vi "LoginInteraction.vi"(10 "LoginStatus":T1, 11 "DataIn":T2={"Quem Joga"="", "Tabuleiro"={"(0,0)"="", "(1,0)"="", "(0,1)"="", "(1,1)"="", "(2,0)"="", "(1,2)"="", "(2,2)"="", "(0,2)"="", "(2,1) "=""}, "GameOption"=enum."Multiplayer local", "Turno"=FALSE, "Player"="", "Player 1"="", "Player 2"="", "Dificuldade"=enum."Easy", "Table"=[], "Row"=0, "Aceitar Convite"=FALSE, "Inviter line"=0, "diretório"=path "", "Logout - panel close"=FALSE, "StartGame"=FALSE, "MatchData.lvclass"=refnum, "GameMode"=enum."Single Easy", "Level State"=FALSE}) -> (2 "Next state":string, 3 "DataOut":T2={"Quem Joga"="", "Tabuleiro"={"(0,0)"="", "(1,0)"="", "(0,1)"="", "(1,1)"="", "(2,0)"="", "(1,2)"="", "(2,2)"="", "(0,2)"="", "(2,1) "=""}, "GameOption"=enum."Multiplayer local", "Turno"=FALSE, "Player"="", "Player 1"="", "Player 2"="", "Dificuldade"=enum."Easy", "Table"=[], "Row"=0, "Aceitar Convite"=FALSE, "Inviter line"=0, "diretório"=path "", "Logout - panel close"=FALSE, "StartGame"=FALSE, "MatchData.lvclass"=refnum, "GameMode"=enum."Single Easy", "Level State"=FALSE})   [LabVIEW 2018]
doc: "SubVI criada para realizar operações de leitura e escrita em arquivo"
uses:
  controls/DataIn.ctl
  MatchDataClasses/MatchData/MatchData.lvclass
  controls/Tabuleiro.ctl
  controls/Table.ctl
  controls/LoginStatus.ctl
  <vilib>/Utility/file.llb/Read Delimited Spreadsheet (string).vi
  <vilib>/Utility/file.llb/Write Delimited Spreadsheet (string).vi
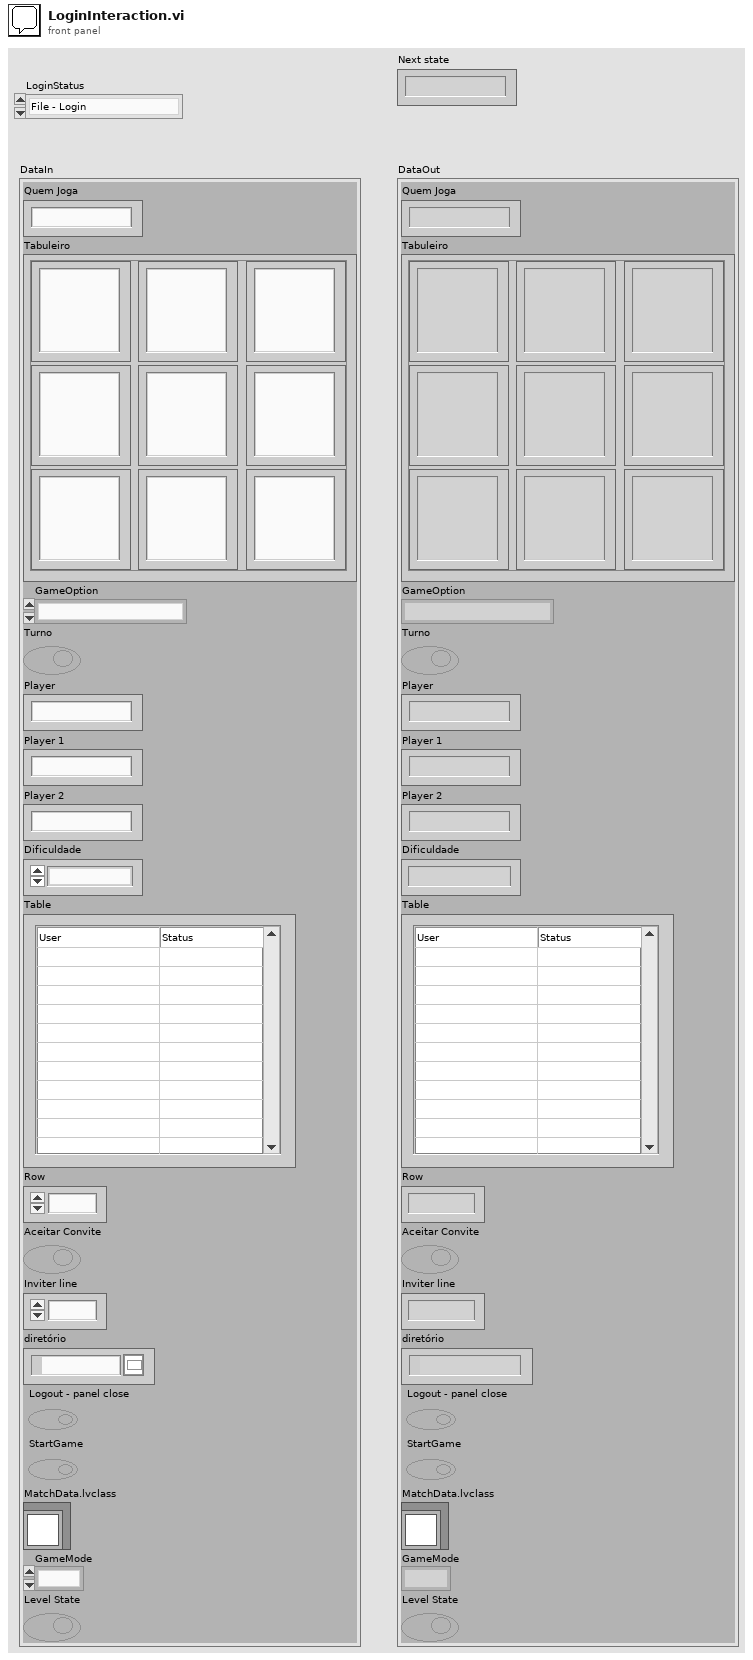
[diagram p1: front panel]
types:
  T1 = typedef "LoginStatus.ctl" = enum16{"File - Login", "File - Logout", "File - TableRefresh"}
  T2 = typedef "DataIn.ctl" = cluster{"Quem Joga":string, "Tabuleiro":T3, "GameOption":enum16{"Single Player", "Multiplayer local", "Multiplayer remoto", "Wait for Event", "Initialize", "Stop"}, "Turno":bool, "Player":string, "Player 1":string, "Player 2":string, "Dificuldade":enum16{"Easy", "Medium", "Hard"}, "Table":T4, "Row":u32, "Aceitar Convite":bool, "Inviter line":u32, "diretório":path, "Logout - panel close":bool, "StartGame":bool, "MatchData.lvclass":refnum<class "MatchData.lvclass">, "GameMode":enum16{"Single Easy", "Single Medium", "Single Hard", "Local", "Remote"}, "Level State":bool}
  T3 = typedef "Tabuleiro.ctl" = cluster{"(0,0)":string, "(1,0)":string, "(0,1)":string, "(1,1)":string, "(2,0)":string, "(1,2)":string, "(2,2)":string, "(0,2)":string, "(2,1) ":string}
  T4 = typedef "Table.ctl" = string[][]
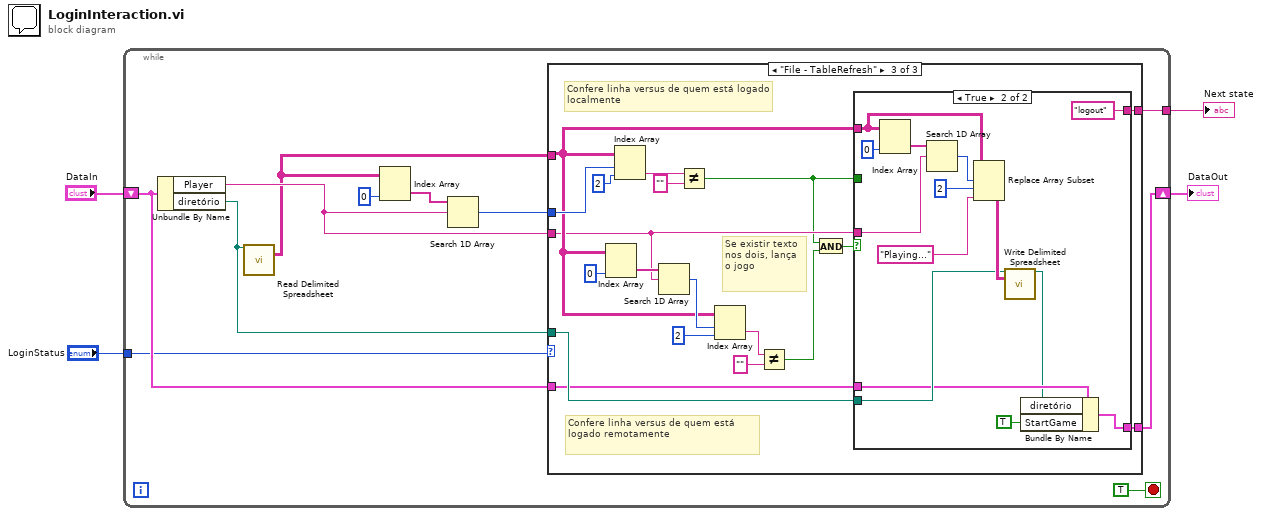
[diagram p0: block diagram]
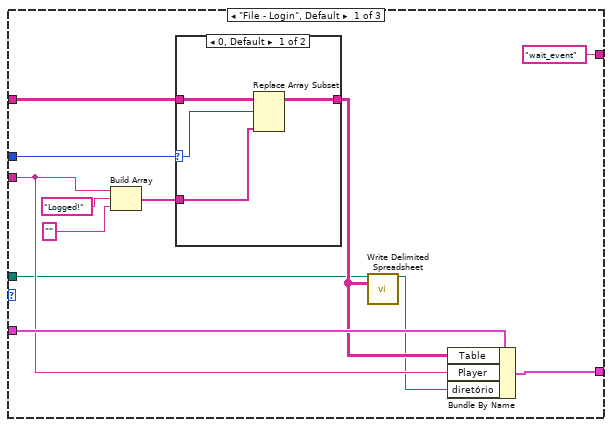
[diagram p2: hidden frame]
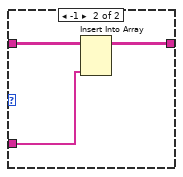
[diagram p3: hidden frame]
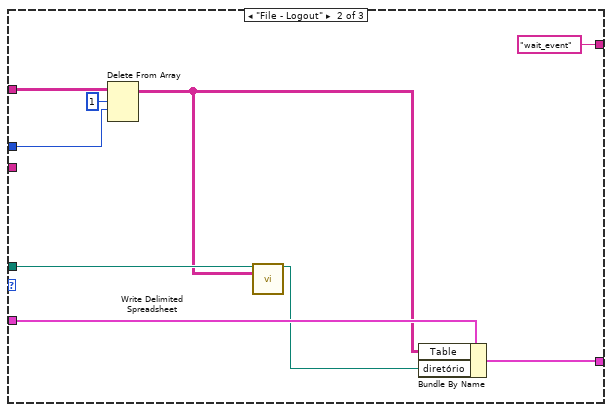
[diagram p4: hidden frame]
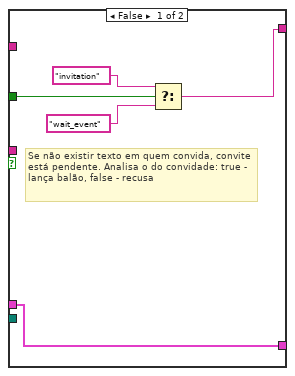
[diagram p5: hidden frame]
diagram:
  n1 = while {
    tunnel: "LoginStatus" -> [w7]
    shift-right: [w8] -> w3
    shift-left: "DataIn" -> [w9]
    tunnel: [w5] -> w1
    stop <- TRUE stop-if-true
    n2 = Unbundle By Name(w9) -> ("Player"=w12:string, "diretório"=w10:path)
    n3 = call-poly <vilib>:"Read Delimited Spreadsheet.vi"("file path (dialog if empty)"=w10) -> ("all rows"=w11:string[][])  [unwired: 9 in, 5 out]
    n4 = Index Array(array=w11, index (col)=0 ("disabled index (col)")) -> (element=w14:string[])  [unwired: 1 in]
    n5 = Search 1D Array(1D array=w14, element=w12) -> (index of element=w13:i32)  [unwired: 1 in]
    n6 = case shown="\"File - TableRefresh\"" w7 {
      tunnel: w13 -> [w25 w42 w62]
      tunnel: w12 -> [w20 _ w49]
      tunnel: w11 -> [w24 w43 w50]
      tunnel: w10 -> [w19 w40 w48]
      tunnel: w9 -> [w22 w39 w47]
      tunnel: [w18 w36 w46] -> w8
      tunnel: ["wait_event" "wait_event" w44] -> w5
      frame "File - Login", Default {
        n7 = Build Array(w20, "Logged!" ("string"), "" ("string")) -> (w23:string[])
        n8 = case shown="0, Default" w25 {
          selector: w25 -> [w30 _]
          tunnel: w23 -> [w28 w32]
          tunnel: w24 -> [w31 w34]
          tunnel: [w29 w33] -> w21
          frame 0, Default {
            n9 = Replace Array Subset(array=w31, new element=w28, index (row)=w30) -> (w29:string[][])  [unwired: 1 in]
          }
          frame -1 {
            n10 = Insert Into Array(array=w34, new element=w32) -> (w33:string[][])  [unwired: 2 in]
          }
        }
        n11 = call-poly <vilib>:"Write Delimited Spreadsheet.vi"("file path (dialog if empty)"=w19, "2D data"=w21) -> ("new file path (Not A Path if cancelled)"=w17:path)  [unwired: 12 in, 1 out]
        n12 = Bundle By Name(cluster=w22, "Table"=w21, "Player"=w20, "diretório"=w17) -> (w18:T2)
      }
      frame "File - Logout" {
        n13 = Delete From Array(array=w43, length=1, index (row)=w42) -> (array with subset deleted=w37:string[][])  [unwired: 1 in, 1 out]
        n14 = call-poly <vilib>:"Write Delimited Spreadsheet.vi"("file path (dialog if empty)"=w40, "2D data"=w37) -> ("new file path (Not A Path if cancelled)"=w38:path)  [unwired: 12 in, 1 out]
        n15 = Bundle By Name(cluster=w39, "Table"=w37, "diretório"=w38) -> (w36:T2)
      }
      frame "File - TableRefresh" {
        # "Confere linha versus de quem está logado localmente"
        # "Confere linha versus de quem está logado remotamente"
        # "Se existir texto nos dois, lança o jogo"
        n16 = Index Array(array=w50, index (col)=0 ("disabled index (col)")) -> (element=w59:string[])  [unwired: 1 in]
        n17 = Index Array(array=w50, index (row)=w62, index (col)=2 ("disabled index (col)")) -> (element=w56:string)
        n18 = Search 1D Array(1D array=w59, element=w49) -> (index of element=w58:i32)  [unwired: 1 in]
        n19 = Not Equal?(x=w56, y="") -> (x != y?=w45:bool)
        n20 = Index Array(array=w50, index (row)=w58, index (col)=2 ("disabled index (col)")) -> (element=w53:string)
        n21 = Not Equal?(x=w53, y="") -> (x != y?=w52:bool)
        n22 = And(x=w45, y=w52) -> (x .and. y?=w51:bool)
        n23 = case shown="True" w51 {
          tunnel: w50 -> [_ w69]
          tunnel: w49 -> [_ w76]
          tunnel: w48 -> [_ w74]
          tunnel: w47 -> [w65 w73]
          tunnel: [w65 w71] -> w46
          tunnel: [w66 "logout"] -> w44
          tunnel: w45 -> [w67 _]
          frame False {
            # "Se não existir texto em quem convida, convite está pendente. Analisa o do convidade: true - lança balão, false - recusa"
            n24 = Select(t="invitation", s=w67, f="wait_event") -> (s? t:f=w66:string)
          }
          frame True {
            n25 = Index Array(array=w69, index (col)=0 ("index (row)")) -> (element=w77:string[])  [unwired: 1 in]
            n26 = Search 1D Array(1D array=w77, element=w76) -> (index of element=w80:i32)  [unwired: 1 in]
            n27 = Replace Array Subset(array=w69, new element="Playing..." ("new element/subarray"), index (row)=w80, index (col)=2 ("disabled index (col)")) -> (w75:string[][])
            n28 = call-poly <vilib>:"Write Delimited Spreadsheet.vi"("file path (dialog if empty)"=w74, "2D data"=w75) -> ("new file path (Not A Path if cancelled)"=w72:path)  [unwired: 12 in, 1 out]
            n29 = Bundle By Name(cluster=w73, "diretório"=w72, "StartGame"=TRUE) -> (w71:T2)
          }
        }
      }
    }
  }
  "DataOut" <- w3
  "Next state" <- w1
